vi "WriteMessage.vi"(8 "error in (no error)":errorcluster, 11 "StepMotor in":refnum<class "StepMotor.lvclass">) -> (0 "error out":errorcluster, 3 "StepMotor out":refnum<class "StepMotor.lvclass">)   [LabVIEW 2010, in "StepMotor.lvclass"]
doc: "Запись сообщения в привод СПШ"
uses:
  StepMotor.lvclass
  StepMotor.lvclass/StepMotor.ctl
panel:
  in  "milliseconds to wait":u32=20
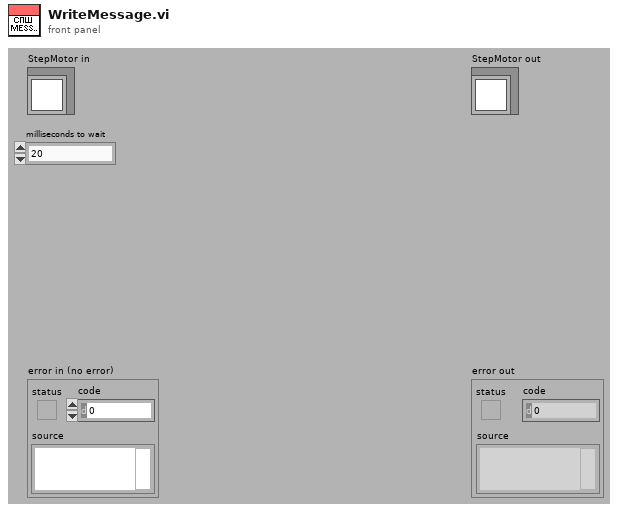
[diagram p1: front panel]
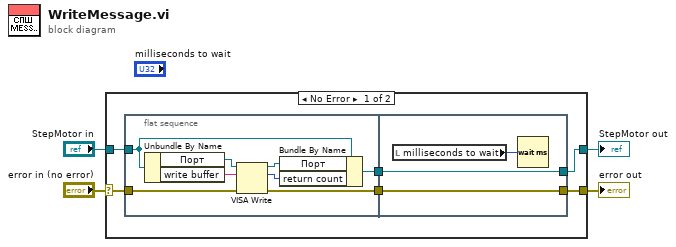
[diagram p0: block diagram]
diagram:
  n1 = case shown="No Error" "error in (no error)" {
    selector: "error in (no error)" -> [w10 w23]
    tunnel: [w7 w23] -> w3
    tunnel: [w9 w22] -> w1
    tunnel: "StepMotor in" -> [w8 w22]
    frame No Error {
      n2 = flat-sequence {
        tunnel: w10 -> [w17]
        tunnel: w8 -> [w15]
        tunnel: [w16] -> w6
        tunnel: [w11] -> w5
        tunnel: [w20] -> w7
        tunnel: [w21] -> w9
        tunnel: w6 -> [w21]
        tunnel: w5 -> [w20]
        frame #0 {
          n3 = Unbundle By Name(w15) -> ("Порт"=w18:refnum<visa-resource-name>, "write buffer"=w14:string)
          n4 = VISA Write(VISA resource name=w18, write buffer=w14, error in (no error)=w17) -> (VISA resource name out=w12:refnum<visa-resource-name>, return count=w13:u32, error out=w11:errorcluster)
          n5 = Bundle By Name(cluster=w15, "Порт"=w12, "return count"=w13) -> (w16:refnum<class "StepMotor.lvclass">)
        }
        frame #1 {
          n6 = local read "milliseconds to wait"() -> (w19:u32)
          n7 = Wait (ms)(milliseconds to wait=w19) -> ()  [unwired: 1 out]
        }
      }
    }
    frame Error {
    }
  }
  "error out" <- w3
  "StepMotor out" <- w1
